vi "Thorlabs-Start Scanning.vi"(8 "error in (no error)":errorcluster, 10 "Tweezertron Ctrl Refs":T1) -> (0 "error out":errorcluster, 2 "Tweezertron Ctrl Refs out":T1, 3 "pDataBuffer":u16[](array[numeric]))   [LabVIEW 2020]
uses:
  _Controls/Tweezertron Ctrl Refs.ctl
  _Controls/Confocal Controls.ctl
  _Controls/iFlex.ctl
  _Controls/PIFOC Position.ctl
  _Controls/Manlight Controls.ctl
  _Controls/Exp Params.ctl
  _Controls/Image Thresholds.ctl
  _Controls/Spots.ctl
  _Globals/pDataBuffer.vi
  ECU_SDK/ThorECU.lvlib
  LSM_SDK/ThorConfocal.lvlib
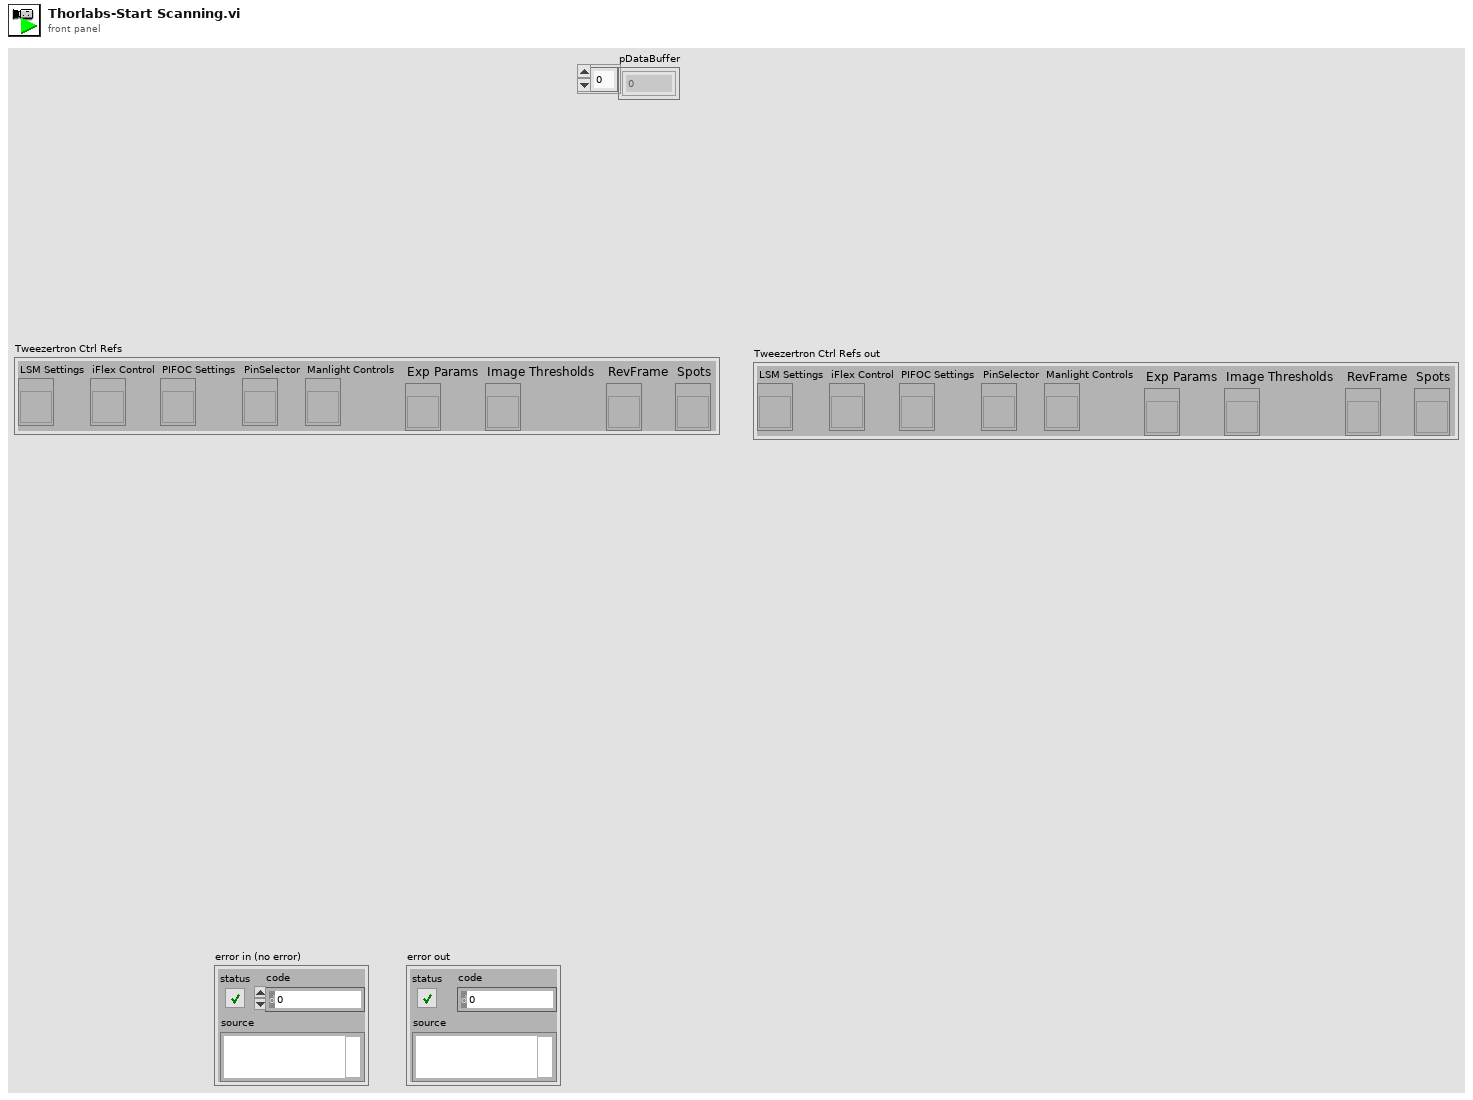
[diagram p1: front panel]
types:
  T1 = typedef "Tweezertron Ctrl Refs.ctl" = cluster{"LSM Settings":refnum<vi>, "iFlex Control":refnum<vi>, "PIFOC Settings":refnum<vi>, "PinSelector":refnum<vi>, "Manlight Controls":refnum<vi>, "Exp Params":refnum<vi>, "Image Thresholds":refnum<vi>, "RevFrame":refnum<vi>, "Spots":refnum<vi>}
  T2 = typedef "Confocal Controls.ctl" = cluster{"Channel Selection":enum32{"A", "B", "AB"}, "Pixel Count":cluster{"Pixels in X":u32, "Pixels in Y":u32}, "Field Size":dbl, "Frames":u8, "Averaging":bool, "Alignment":dbl, "Scan Mode":bool, "Gain":cluster{"Gain A":u8, "Gain B":u8}, "Enable PMTs":cluster{"A":bool, "B":bool}, "Voltage Range":cluster{"Range A":u16, "Range B":u16}, "Multi Frame Count":dbl, "Trigger Mode":dbl, "Real Time Averaging":bool, "PFOV":dbl, "MicronsPerPx":dbl}
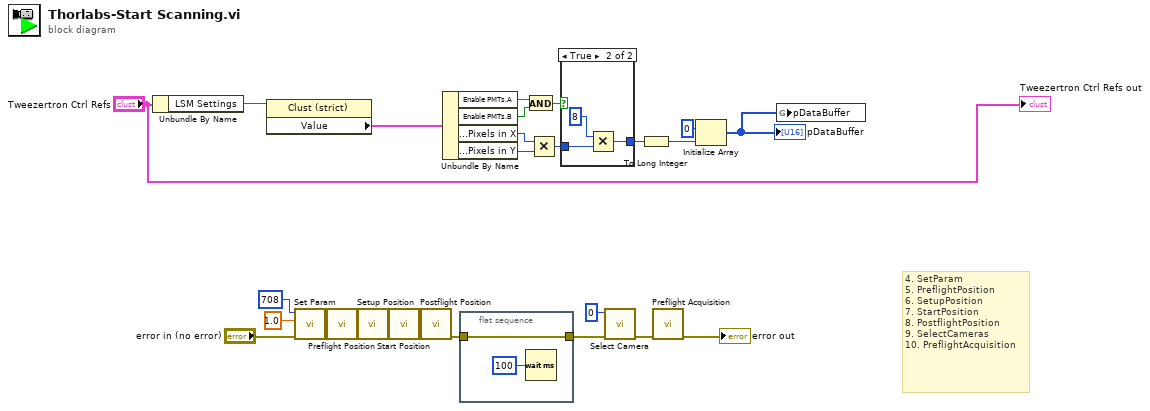
[diagram p0: block diagram]
diagram:
  # "4. SetParam\n5. PreflightPosition\n6. SetupPosition\n7. StartPosition\n8. PostflightPosition\n9. SelectCameras\n10. PreflightAcquisition"
  n1 = Unbundle By Name("Tweezertron Ctrl Refs") -> ("LSM Settings"=w2:refnum<vi>)
  n2 = property class="Clust (strict)"(reference=w2) -> ("Value"=w1:T2)  [unwired: 1 in, 2 out]
  n3 = call "Set Param.vi"("error in (no error)"="error in (no error)", "param"=1.0, "paramID"=708) -> ("error out"=w23:errorcluster)  [unwired: 7 in, 1 out]
  n4 = call "Preflight Position.vi"("error in (no error)"=w23) -> ("error out"=w22:errorcluster)  [unwired: 9 in, 1 out]
  n5 = call "Setup Position.vi"("error in (no error)"=w22) -> ("error out"=w21:errorcluster)  [unwired: 9 in, 1 out]
  n6 = call "Start Position.vi"("error in (no error)"=w21) -> ("error out"=w19:errorcluster)  [unwired: 9 in, 1 out]
  n7 = call "Postflight Position.vi"("error in (no error)"=w19) -> ("error out"=w14:errorcluster)  [unwired: 9 in, 1 out]
  n8 = Unbundle By Name(w1) -> ("Enable PMTs.A"=w7:bool, "Enable PMTs.B"=w8:bool, "Pixel Count.Pixels in X"=w6:u32, "Pixel Count.Pixels in Y"=w9:u32)
  n9 = flat-sequence {
    tunnel: [w27] -> w15
    tunnel: w14 -> [w27]
    frame #0 {
      n10 = Wait (ms)(milliseconds to wait=u32 100) -> ()  [unwired: 1 out]
    }
  }
  n11 = And(x=w7, y=w8) -> (x .and. y?=w13:bool)
  n12 = Multiply(x=w6, y=w9) -> (x*y=w10:u32)
  n13 = case shown="True" w13 {
    tunnel: w10 -> [w28 w31]
    tunnel: [w28 w29] -> w12
    frame False {
    }
    frame True {
      n14 = Multiply(x=u32 8, y=w31) -> (x*y=w29:u32)
    }
  }
  n15 = call "Select Camera.vi"("error in (no error)"=w15, "camera"=0) -> ("error out"=w17:errorcluster)  [unwired: 4 in, 1 out]
  n16 = To Long Integer(number=w12) -> (32bit integer=w5:i32)
  n17 = call "Preflight Acquisition.vi"("error in (no error)"=w17) -> ("error out"=→"error out":errorcluster)  [unwired: 4 in, 2 out]
  n18 = Initialize Array(u16 0, w5) -> (w4:u16[])
  "pDataBuffer" <- w4
  n19 = global write "pDataBuffer.vi" "pDataBuffer"(w4) -> ()
  "Tweezertron Ctrl Refs out" <- "Tweezertron Ctrl Refs"
